vi "Stalker.vi"(8 "Error In":errorcluster, 11 "Refnum's In":T1={"Gyro"="Gyro", "Mtr 1"="LeftMtr", "Mtr 2"="RightMtr"}) -> (0 "Error Out":errorcluster, 3 "Refnum's Out":T1={"Gyro"="Gyro", "Mtr 1"="LeftMtr", "Mtr 2"="RightMtr"})   [LabVIEW 2016]
uses:
  Robot Global Data.vi
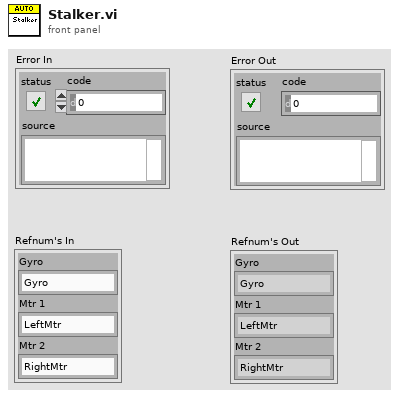
[diagram p1: front panel]
types:
  T1 = cluster{"Gyro":string, "Mtr 1":string, "Mtr 2":string}
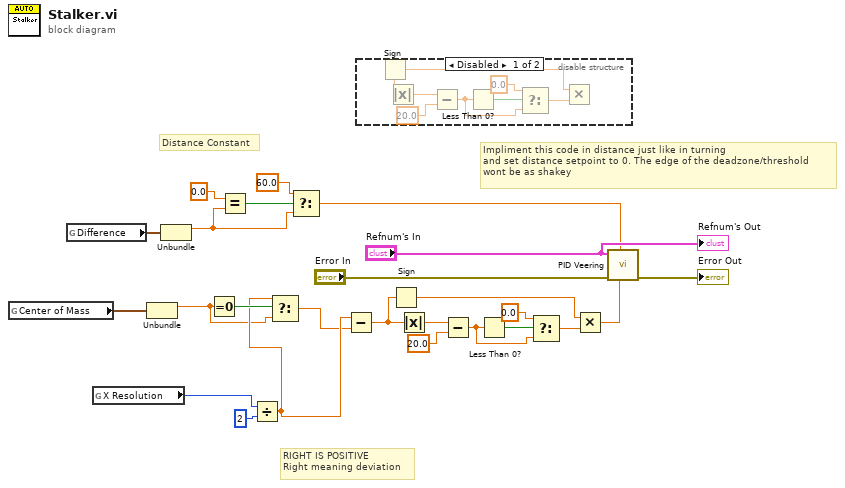
[diagram p0: block diagram]
diagram:
  # "Impliment this code in distance just like in turning\nand set distance setpoint to 0. The edge of the deadzone/threshold\nwont be as shakey"
  # "Distance Constant"
  # "RIGHT IS POSITIVE\nRight meaning deviation"
  n1 = global read "Robot Global Data.vi" "Center of Mass"() -> (w23:cluster{"X":dbl, "Y":dbl})
  n2 = global read "Robot Global Data.vi" "Difference"() -> (w11:cluster{"X":dbl, "Y":dbl})
  n3 = global read "Robot Global Data.vi" "X Resolution"() -> (w21:i32)
  n4 = Unbundle(w23) -> ("X"=w13:dbl)  [unwired: 1 out]
  n5 = Unbundle(w11) -> ("X"=w10:dbl)  [unwired: 1 out]
  n6 = Equal To 0?(x=w13) -> (x = 0?=w15:bool)
  n7 = Equal?(x=0.0 ("y"), y=w10) -> (x = y?=w19:bool)
  n8 = Divide(x=w21, y=2) -> (x/y=w14:dbl)
  n9 = Select(t=w14, s=w15, f=w13) -> (s? t:f=w12:dbl)
  n10 = Select(t=60.0 ("x"), s=w19, f=w10) -> (s? t:f=w16:dbl)
  n11 = Subtract(x=w14, y=w12) -> (x-y=w4:dbl)
  n12 = disable-structure shown="Disabled" {
    frame Disabled {
      n13 = Absolute Value() -> (x=w28:dbl, abs(x)=w33:dbl)
      n14 = Sign(1:w28) -> (0:w26:dbl)
      n15 = Subtract(x=w33, y=20.0) -> (x-y=w29:dbl)
      n16 = Less Than 0?(x=w29) -> (x < 0?=w31:bool)
      n17 = Select(t=0.0, s=w31, f=w29) -> (s? t:f=w27:dbl)
      n18 = Multiply(x=w26, y=w27) -> ()  [unwired: 1 out]
    }
    frame Enabled {
    }
  }
  n19 = Sign(1:w4) -> (0:w2:dbl)
  n20 = Absolute Value(x=w4) -> (abs(x)=w9:dbl)
  n21 = Subtract(x=w9, y=20.0) -> (x-y=w5:dbl)
  n22 = Less Than 0?(x=w5) -> (x < 0?=w7:bool)
  n23 = Select(t=0.0, s=w7, f=w5) -> (s? t:f=w3:dbl)
  n24 = Multiply(x=w2, y=w3) -> (x*y=w1:dbl)
  n25 = call "PID Veering.vi"("Deviation"=w1, "Current Distance"=w16, "error in (no error)"="Error In", "Refnum's"="Refnum's In") -> ("error out"=→"Error Out":errorcluster)  [unwired: 7 in]
  "Refnum's Out" <- "Refnum's In"
